vi "FGVScanParameters.vi"(7 "Enum":T2, 8 "error in":errorcluster, 9 "Scan Parameters In":T1={"Width"=0.0, "Height"=0.0, "X Offset"=0.0, "Y Offset"=0.0, "Angle"=0.0, "Pixels/Line"=2, "Lines"=0, "Time/Line"=0.0, "Scan Rate"=0.0} {"Scan Rate" format="%.2fHz"; "Lines" format="%#.0f"; "Pixels/Line" min=2 max=8192 format="%#.0f"; "Height" format="%#_6pm"; "Width" format="%#_6pm"; "Time/Line" format="%.2ps"; "Angle" format="%.2f°"; "Y Offset" format="%#_6pm"; "X Offset" format="%#_6pm"}) -> (0 "error out":errorcluster, 1 "Scan Parameters Out":T1={"Width"=0.0, "Height"=0.0, "X Offset"=0.0, "Y Offset"=0.0, "Angle"=0.0, "Pixels/Line"=2, "Lines"=0, "Time/Line"=0.0, "Scan Rate"=0.0} {"Scan Rate" format="%.2fHz"; "Lines" format="%#.0f"; "Pixels/Line" min=2 max=8192 format="%#.0f"; "Height" format="%#_6pm"; "Width" format="%#_6pm"; "Time/Line" format="%.2ps"; "Angle" format="%.2f°"; "Y Offset" format="%#_6pm"; "X Offset" format="%#_6pm"})   [LabVIEW 2016]
uses:
  controls/Enum.ctl
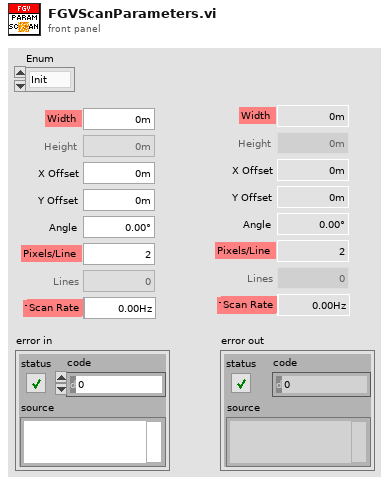
[diagram p1: front panel]
types:
  T1 = cluster{"Width":dbl, "Height":dbl, "X Offset":dbl, "Y Offset":dbl, "Angle":dbl, "Pixels/Line":u16, "Lines":u16, "Time/Line":dbl, "Scan Rate":dbl}
  T2 = typedef "Enum.ctl" = enum16{"Init", "Read", "Write"}
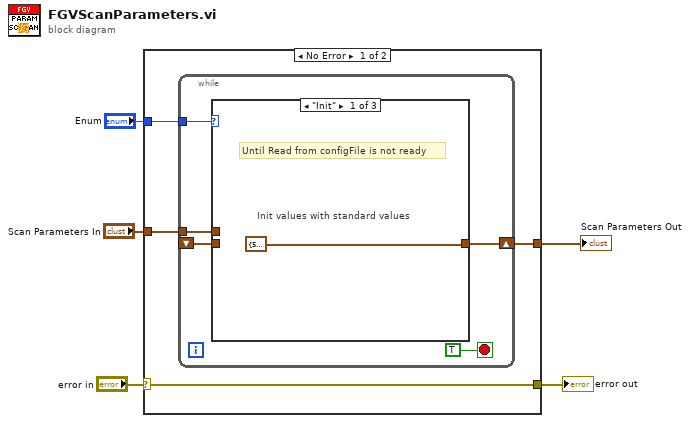
[diagram p0: block diagram]
diagram:
  n1 = case shown="No Error" "error in" {
    selector: "error in" -> [w8 w19]
    tunnel: "Enum" -> [w9 _]
    tunnel: [w8 w19] -> w4
    tunnel: "Scan Parameters In" -> [w7 w18]
    tunnel: [w6 w18] -> w1
    frame No Error {
      n2 = while {
        tunnel: w9 -> [w13]
        tunnel: w7 -> [w12]
        shift-right: [w11] -> w6
        shift-left: _ -> [w10]
        stop <- TRUE stop-if-true
        n3 = case shown="\"Init\"" w13 {
          tunnel: w12 -> [_ _ w17]
          tunnel: [T1 {"Width"=5e-07, "Height"=5e-07, "X Offset"=0.0, "Y Offset"=0.0, "Angle"=0.0, "Pixels/Line"=256, "Lines"=256, "Time/Line"=1.0, "Scan Rate"=1.0} ("Scan Parameters In") w16 w17] -> w11
          tunnel: w10 -> [_ w16 _]
          frame "Init" {
            # "Init values with standard values"
            # "Until Read from configFile is not ready"
          }
          frame "Read", Default {
          }
          frame "Write" {
          }
        }
      }
    }
    frame Error {
    }
  }
  "error out" <- w4
  "Scan Parameters Out" <- w1
